vi "PMC_TESTER_Working_V2.vi"() -> ()   [LabVIEW 2018]
uses:
  <vilib>/ptbypt/NI_PtbyPt.lvlib
  <vilib>/Utility/file.llb/Write Delimited Spreadsheet (string).vi
panel:
  in  "PMC thickness (m)":string
  in  "PMC Area (m^2)":string
  out "K_B":string
  out "K_A":string
  out "Delta_B (T2 - T3)":string
  out "Delta_A (T0 - T1)":string
  in  "Heater Resistance (Ohm)":string
  out "Required Voltage Setting":string
  in  "Power Input (W)":string
  in  "Quit":bool
  in  "Number of Samples":string
  out "Output Preview (C)":string[][](array[string])
  out "Current Sample Averages (C)":string[](array[string])
  in  "Frequency (hz)":string
  in  "Stop Data Acquisition":bool
  out "Runtime (s)":string
  in  "Export Button":bool
  in  "Time Increment (s)":string
  out "Live Temperature Data":dynamicdata(graph)
  # "SAMPLING"
  # "SAMPLE PROPERTIES"
  # "PMC TESTER"
  # "Aaron Scott - Spring 2020"
  # "Ambient"
  # "T0"
  # "T1"
  # "T2"
  # "T3"
  # "K_A"
  # "K_B"
  # "Time"
  # "Ambient"
  # "T0"
  # "T1"
  # "T2"
  # "T3"
  # "K_A"
  # "K_B"
  # "Time"
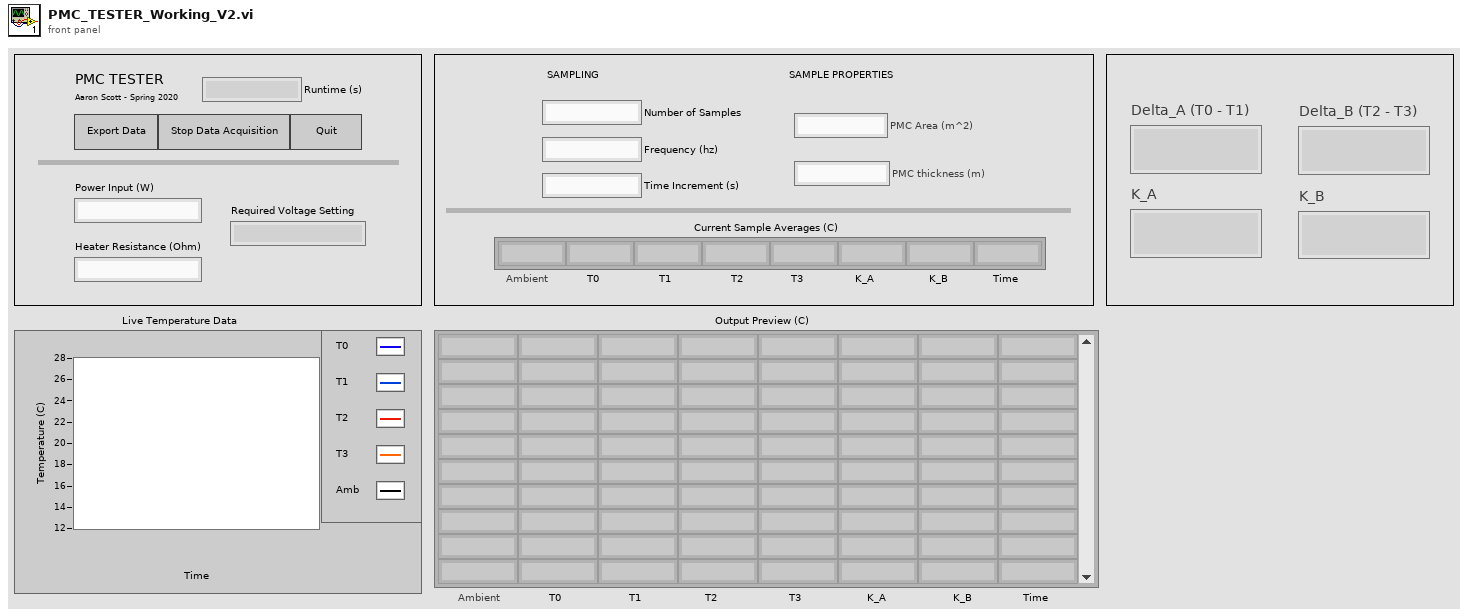
[diagram p1: front panel]
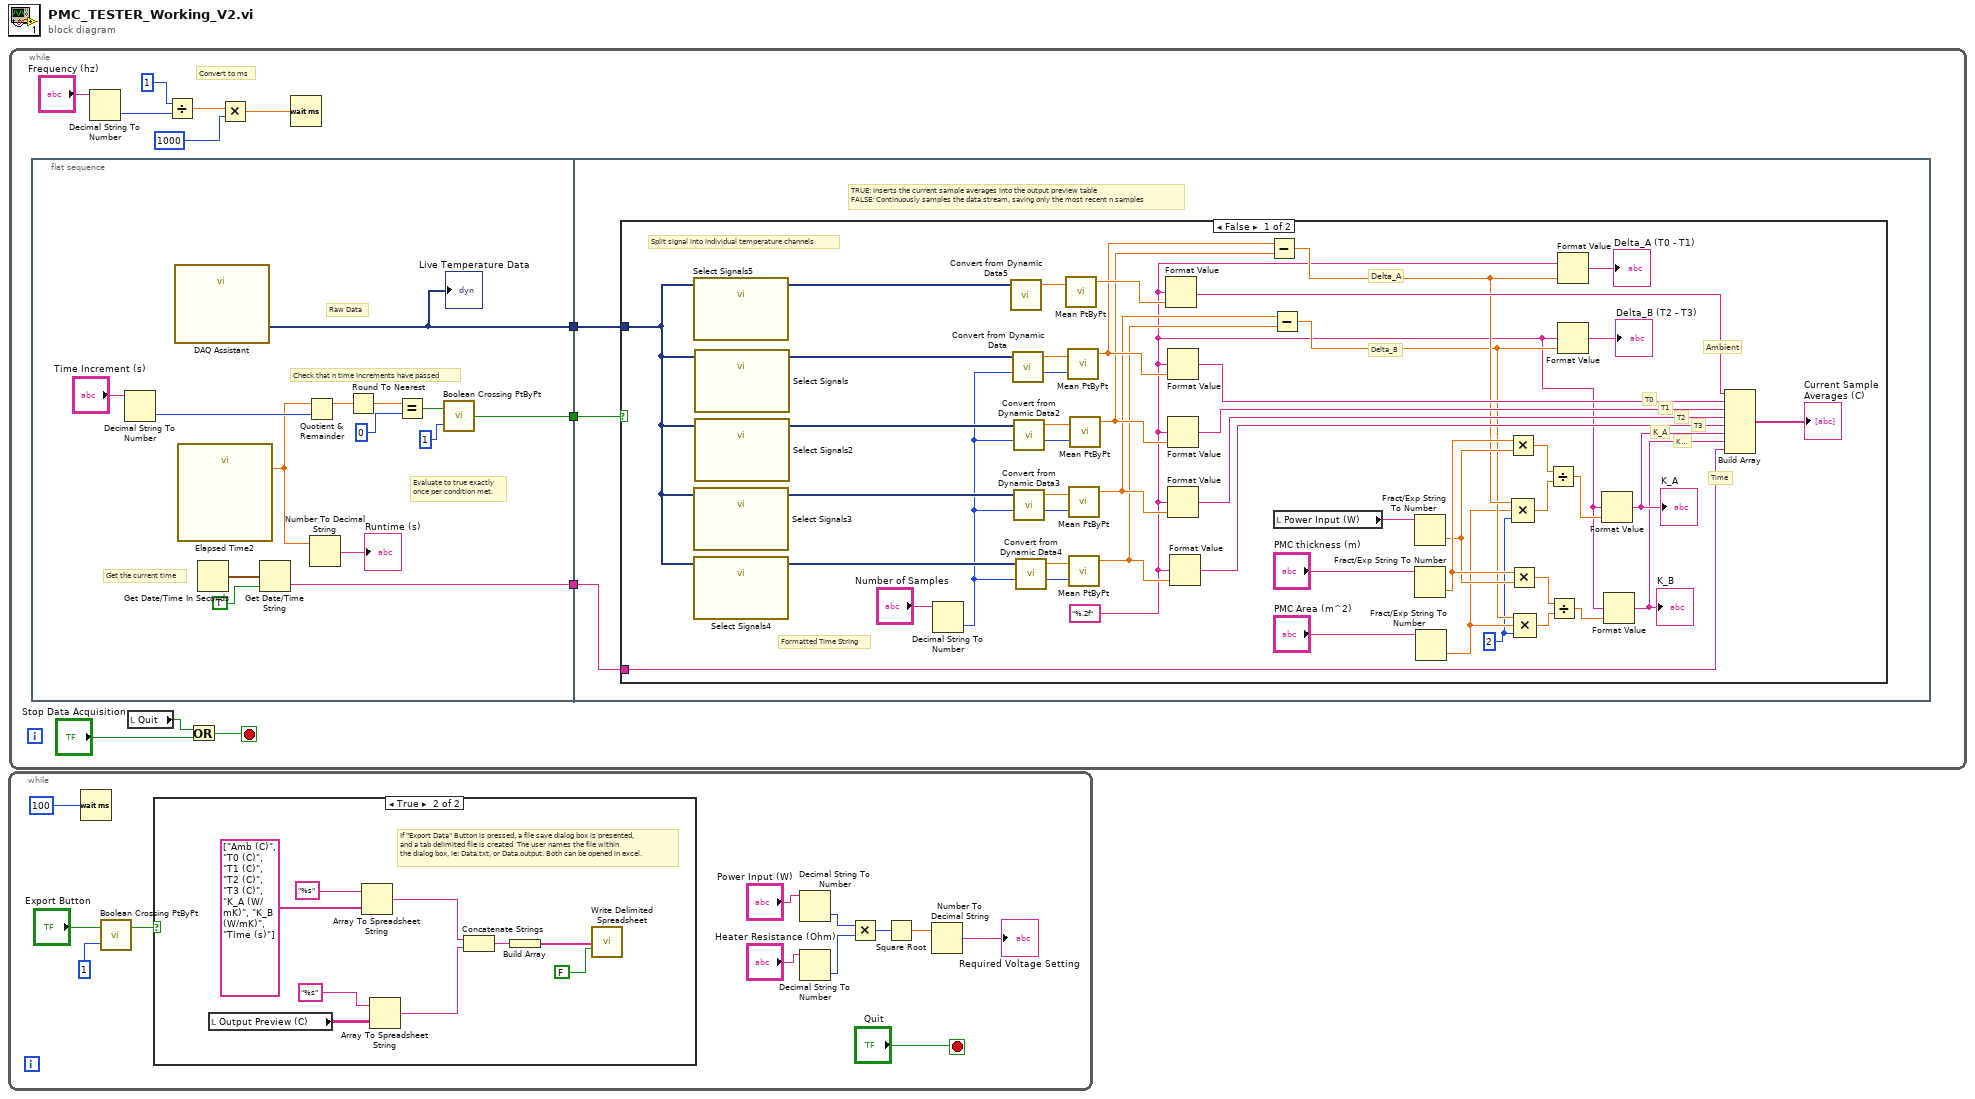
[diagram p0: block diagram]
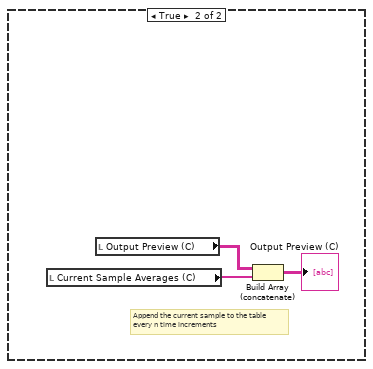
[diagram p3: hidden frame]
diagram:
  n1 = while {
    stop <- "Quit" stop-if-true
    n2 = Wait (ms)(milliseconds to wait=100) -> ()  [unwired: 1 out]
    n3 = call <vilib>:"Boolean Crossing PtByPt.vi"("direction"=1, "input"="Export Button") -> ("crossing"=w11:bool)  [unwired: 1 in]
    n4 = case shown="True" w11 {
      frame False {
      }
      frame True {
        # "If \"Export Data\" Button is pressed, a file save dialog box is presented,\nand a tab delimited file is created. The user names the file within \nthe dialog box, ie: Data.txt, or Data.output. Both can be opened in excel."
        n5 = local read "Output Preview (C)"() -> (w21:string[][])
        n6 = Array To Spreadsheet String(array=string[] ["Amb (C)", "T0 (C)", "T1 (C)", "T2 (C)", "T3 (C)", "K_A (W/mK)", "K_B (W/mK)", "Time (s)"], 3:"%s") -> (spreadsheet string=w15:string)  [unwired: 1 in]
        n7 = Array To Spreadsheet String(array=w21, 3:"%s") -> (spreadsheet string=w14:string)  [unwired: 1 in]
        n8 = Concatenate Strings(w15, w14) -> (w18:string)
        n9 = Build Array(w18) -> (w17:string[])
        n10 = call-poly <vilib>:"Write Delimited Spreadsheet.vi"("1D data"=w17, "append to file? (new file:F)"=FALSE) -> ()  [unwired: 12 in, 2 out]
      }
    }
    n11 = Decimal String To Number(string="Power Input (W)") -> (number=w5:i32)  [unwired: 2 in, 1 out]
    n12 = Decimal String To Number(string="Heater Resistance (Ohm)") -> (number=w4:i32)  [unwired: 2 in, 1 out]
    n13 = Multiply(x=w5, y=w4) -> (x*y=w3:i32)
    n14 = Square Root(x=w3) -> (sqrt(x)=w2:dbl)
    n15 = Number To Decimal String(number=w2) -> (decimal integer string=→"Required Voltage Setting":string)  [unwired: 1 in]
  }
  n16 = while {
    stop <- w23 stop-if-true
    # "Convert to ms"
    n17 = flat-sequence {
      tunnel: [w37] -> w33
      tunnel: [w40] -> w32
      tunnel: [w35] -> w22
      tunnel: w33 -> [w50]
      tunnel: w32 -> [w49]
      tunnel: w22 -> [w48]
      frame #0 {
        # "Get the current time"
        # "Raw Data"
        # "Evaluate to true exactly\nonce per condition met."
        # "Check that n time increments have passed"
        n18 = Decimal String To Number(string="Time Increment (s)") -> (number=w42:i32)  [unwired: 2 in, 1 out]
        n19 = call "DAQ Assistant"() -> ("data"=w37:dynamicdata)  [unwired: 17 in, 2 out]
        "Live Temperature Data" <- w37
        n20 = call "Elapsed Time2"() -> ("Elapsed Time (s)"=w38:dbl)  [unwired: 12 in, 7 out]
        n21 = Get Date/Time In Seconds() -> (seconds since 1Jan1904=w36:timestamp)
        n22 = Get Date/Time String(seconds (now)=w36, want seconds? (F)=TRUE) -> (time string=w35:string)  [unwired: 1 in, 1 out]
        n23 = Quotient & Remainder(x=w38, y=w42) -> (x-y*floor(x/y)=w45:dbl)  [unwired: 1 out]
        n24 = Number To Decimal String(number=w38) -> (decimal integer string=→"Runtime (s)":string)  [unwired: 1 in]
        n25 = Round To Nearest(number=w45) -> (nearest integer value=w46:dbl)
        n26 = Equal?(x=w46, y=0) -> (x = y?=w41:bool)
        n27 = call <vilib>:"Boolean Crossing PtByPt.vi"("direction"=1, "input"=w41) -> ("crossing"=w40:bool)  [unwired: 1 in]
      }
      frame #1 {
        # "TRUE: Inserts the current sample averages into the output preview table\nFALSE: Continuously samples the data stream, saving only the most recent n samples"
        n28 = case shown="False" w49 {
          tunnel: w50 -> [w77 _]
          tunnel: w48 -> [w54 _]
          frame False {
            w51 = 2
            w55 = "%.2f"
            # "Time"
            # "K_B"
            # "K_A"
            # "Delta_B"
            # "Delta_A"
            # "Ambient"
            # "T3"
            # "T2"
            # "T1"
            # "T0"
            # "Formatted Time String"
            # "Split signal into individual temperature channels"
            n29 = call "Select Signals5"("Signals"=w77) -> ("Signal Out"=w76:dynamicdata)  [unwired: 9 in, 1 out]
            n30 = call "Select Signals3"("Signals"=w77) -> ("Signal Out"=w93:dynamicdata)  [unwired: 9 in, 1 out]
            n31 = call "Select Signals4"("Signals"=w77) -> ("Signal Out"=w92:dynamicdata)  [unwired: 9 in, 1 out]
            n32 = call "Select Signals"("Signals"=w77) -> ("Signal Out"=w95:dynamicdata)  [unwired: 9 in, 1 out]
            n33 = call "Select Signals2"("Signals"=w77) -> ("Signal Out"=w94:dynamicdata)  [unwired: 9 in, 1 out]
            n34 = Decimal String To Number(string="Number of Samples") -> (number=w86:i32)  [unwired: 2 in, 1 out]
            n35 = call "Convert from Dynamic Data5"("Dynamic Data Type"=w76) -> ("Scalar"=w80:dbl)  [unwired: 3 in]
            n36 = call "Convert from Dynamic Data"("Dynamic Data Type"=w95) -> ("Scalar"=w91:dbl)  [unwired: 3 in]
            n37 = call "Convert from Dynamic Data2"("Dynamic Data Type"=w94) -> ("Scalar"=w90:dbl)  [unwired: 3 in]
            n38 = call "Convert from Dynamic Data3"("Dynamic Data Type"=w93) -> ("Scalar"=w89:dbl)  [unwired: 3 in]
            n39 = call "Convert from Dynamic Data4"("Dynamic Data Type"=w92) -> ("Scalar"=w88:dbl)  [unwired: 3 in]
            n40 = call <vilib>:"Mean PtByPt.vi"("x"=w80) -> ("mean"=w79:dbl)  [unwired: 3 in, 1 out]
            n41 = call <vilib>:"Mean PtByPt.vi"("x"=w91, "sample length"=w86) -> ("mean"=w75:dbl)  [unwired: 2 in, 1 out]
            n42 = call <vilib>:"Mean PtByPt.vi"("x"=w89, "sample length"=w86) -> ("mean"=w73:dbl)  [unwired: 2 in, 1 out]
            n43 = call <vilib>:"Mean PtByPt.vi"("x"=w88, "sample length"=w86) -> ("mean"=w72:dbl)  [unwired: 2 in, 1 out]
            n44 = call <vilib>:"Mean PtByPt.vi"("x"=w90, "sample length"=w86) -> ("mean"=w74:dbl)  [unwired: 2 in, 1 out]
            n45 = Format Value(format string=w55, value (0)=w79) -> (output string=w78:string)  [unwired: 1 in]
            n46 = Format Value(format string=w55, value (0)=w75) -> (output string=w81:string)  [unwired: 1 in]
            n47 = Format Value(format string=w55, value (0)=w74) -> (output string=w82:string)  [unwired: 1 in]
            n48 = Format Value(format string=w55, value (0)=w73) -> (output string=w83:string)  [unwired: 1 in]
            n49 = Format Value(format string=w55, value (0)=w72) -> (output string=w84:string)  [unwired: 1 in]
            n50 = Subtract(x=w75, y=w74) -> (x-y=w64:dbl)
            n51 = Subtract(x=w73, y=w72) -> (x-y=w63:dbl)
            n52 = local read "Power Input (W)"() -> (w69:string)
            n53 = Fract/Exp String To Number(string=w69) -> (number=w65:dbl)  [unwired: 3 in, 1 out]
            n54 = Fract/Exp String To Number(string="PMC thickness (m)") -> (number=w66:dbl)  [unwired: 3 in, 1 out]
            n55 = Fract/Exp String To Number(string="PMC Area (m^2)") -> (number=w62:dbl)  [unwired: 3 in, 1 out]
            n56 = Multiply(x=w66, y=w65) -> (x*y=w59:dbl)
            n57 = Multiply(x=w66, y=w65) -> (x*y=w61:dbl)
            n58 = Compound Arithmetic op=MULTIPLY(w64, w62, w51) -> (w58:dbl)
            n59 = Compound Arithmetic op=MULTIPLY(w63, w62, w51) -> (w60:dbl)
            n60 = Divide(x=w59, y=w58) -> (x/y=w57:dbl)
            n61 = Divide(x=w61, y=w60) -> (x/y=w56:dbl)
            n62 = Format Value(format string=w55, value (0)=w64) -> (output string=→"Delta_A (T0 - T1)":string)  [unwired: 1 in]
            n63 = Format Value(format string=w55, value (0)=w63) -> (output string=→"Delta_B (T2 - T3)":string)  [unwired: 1 in]
            n64 = Format Value(format string=w55, value (0)=w57) -> (output string=w53:string)  [unwired: 1 in]
            "K_A" <- w53
            n65 = Format Value(format string=w55, value (0)=w56) -> (output string=w52:string)  [unwired: 1 in]
            "K_B" <- w52
            n66 = Build Array(w78, w81, w82, w83, w84, w53, w52, w54) -> (→"Current Sample Averages (C)":string[])
          }
          frame True {
            # "Append the current sample to the table\nevery n time increments"
            n67 = local read "Current Sample Averages (C)"() -> (w96:string[])
            n68 = local read "Output Preview (C)"() -> (w98:string[][])
            n69 = Build Array (concatenate)(w98, w96) -> (→"Output Preview (C)":string[][])
          }
        }
      }
    }
    n70 = Decimal String To Number(string="Frequency (hz)") -> (number=w29:i32)  [unwired: 2 in, 1 out]
    n71 = local read "Quit"() -> (w25:bool)
    n72 = Divide(x=1, y=w29) -> (x/y=w27:dbl)
    n73 = Or(x=w25, y="Stop Data Acquisition") -> (x .or. y?=w23:bool)
    n74 = Multiply(x=w27, y=1000) -> (x*y=w26:dbl)
    n75 = Wait (ms)(milliseconds to wait=w26) -> ()  [unwired: 1 out]
  }
